vi "Matrix_Diag.vi"(11 "input matrix":T1) -> (3 "output matrix":T1)   [LabVIEW 2019, in "Trajectory_Library.lvlib"]
doc: "Returns the diagonal elements inside a vector or square matrix.\n \nIf \"this\" Matrix is a vector then a square matrix is returned. If a \"this\" Matrix}is a matrix then a vector of diagonal elements is returned.\n \n\nInputs:\n - input matrix -- The input matrix\n\nOutputs:\n - output matrix -- The diagonal elements inside a vector or a square matrix."
uses:
  Trajectory_Library.lvlib
  <vilib>/Analysis/Matrix/Datatypes/RealMatrix.ctl
  <vilib>/Analysis/Matrix/NI_Matrix.lvlib
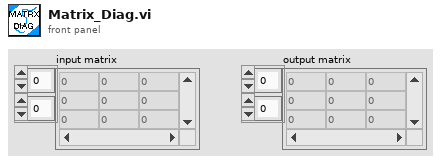
[diagram p1: front panel]
types:
  T1 = typedef "NI_Matrix.lvlib/RealMatrix.ctl" = dbl[][]
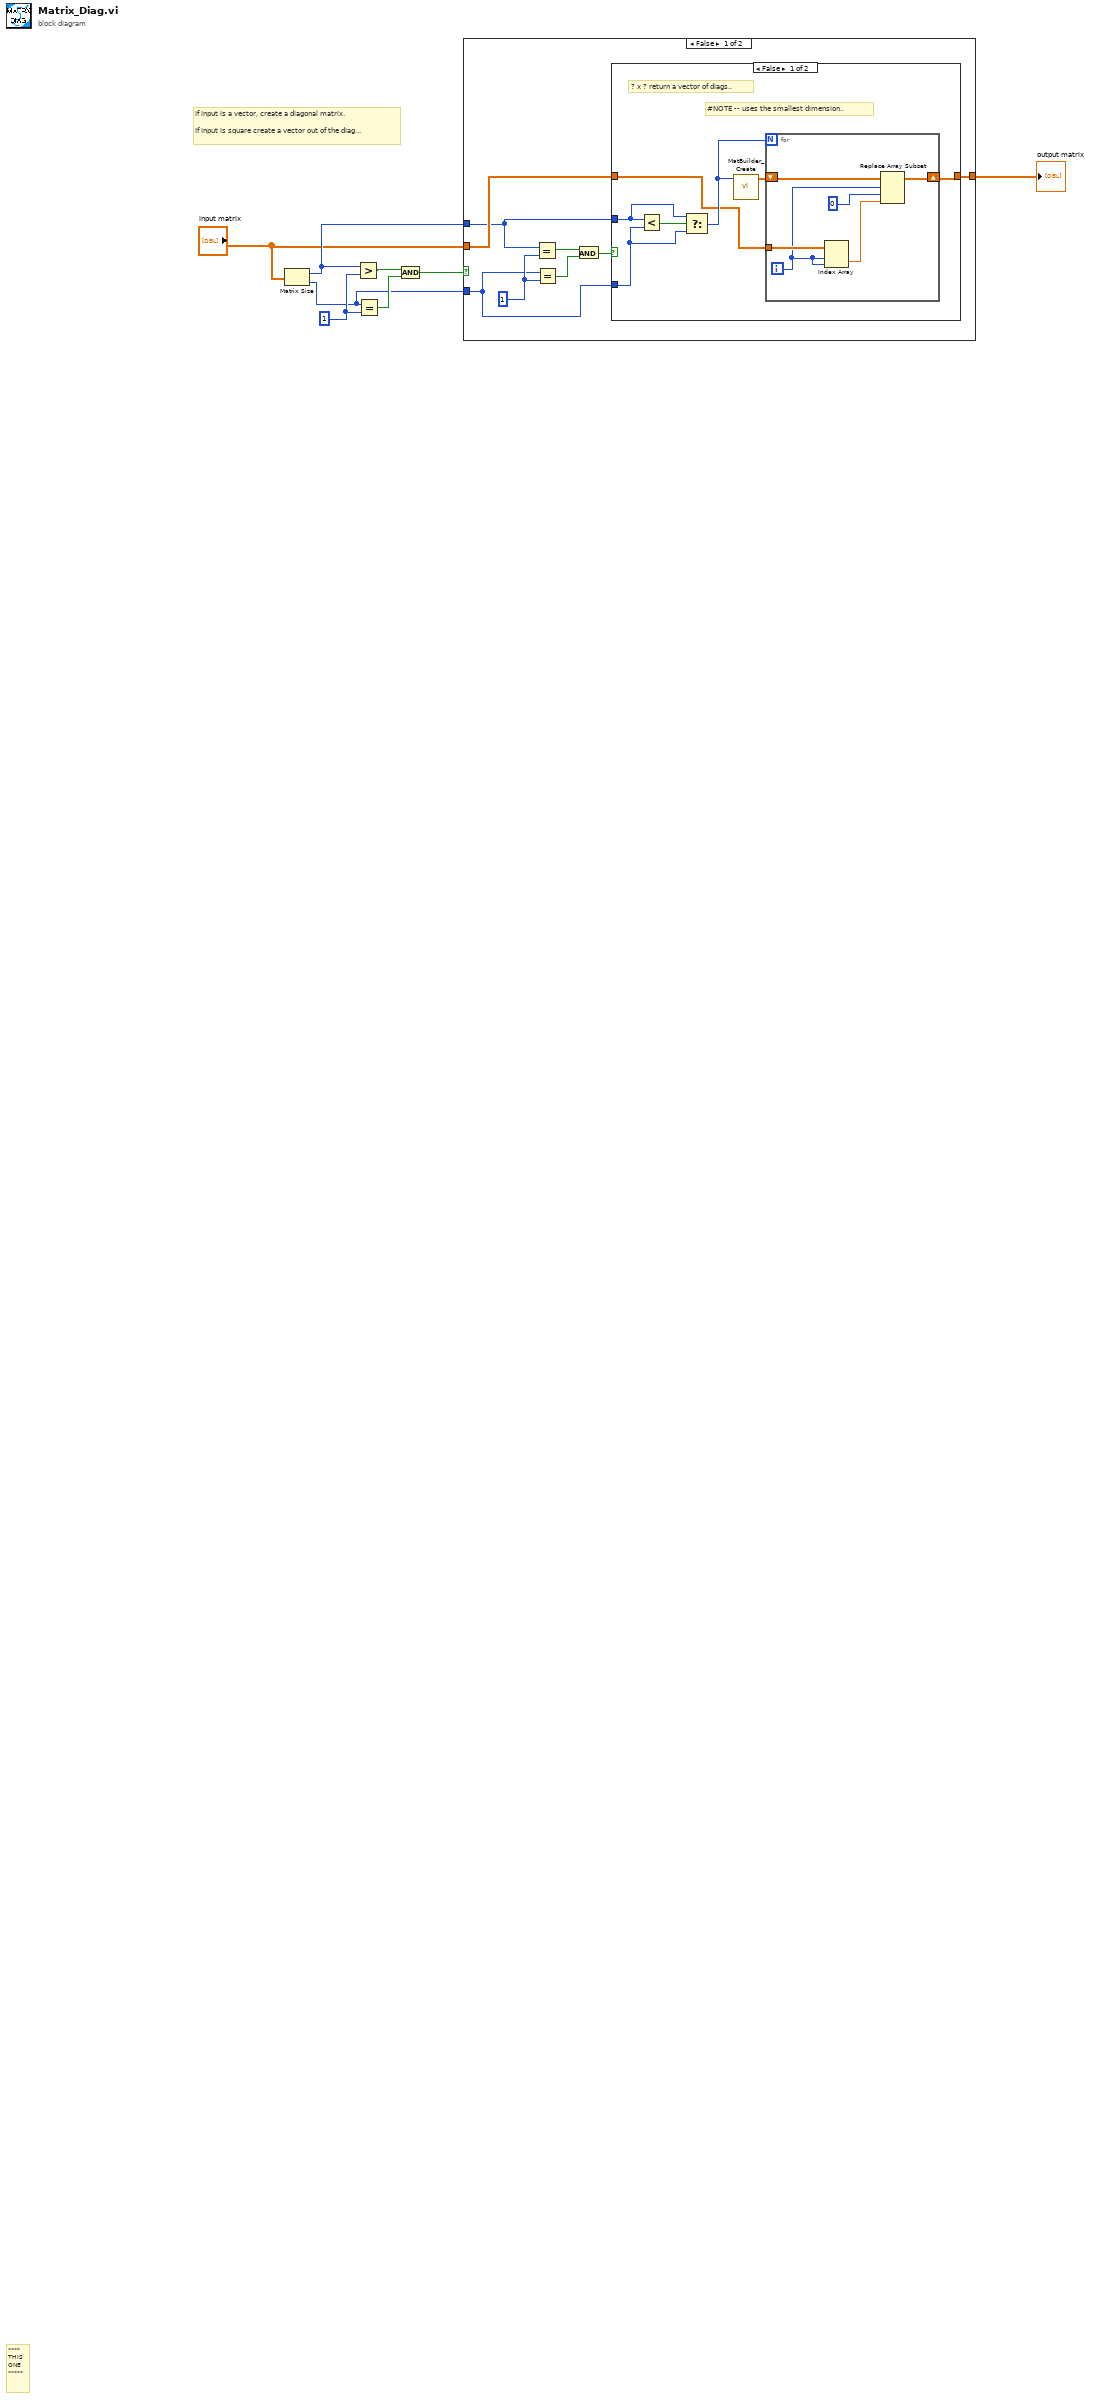
[diagram p0: block diagram]
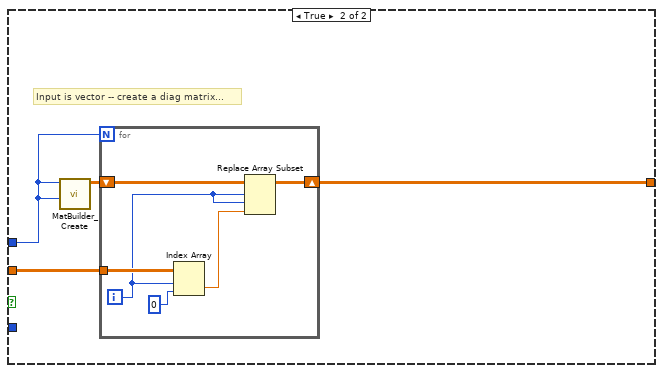
[diagram p3: hidden frame]
diagram:
  w8 = 1 ("y")
  # "If input is a vector, create a diagonal matrix.  \n\nIf input is square create a vector out of the diag..."
  # "****\nTHIS\nONE\n*****"
  n1 = Matrix Size(0:"input matrix") -> (1:w4:i32, 2:w1:i32)
  n2 = Greater?(x=w4, y=w8) -> (0:w7:bool)
  n3 = Equal?(x=w1, y=w8) -> (x = y?=w6:bool)
  n4 = And(x=w7, y=w6) -> (x .and. y?=w5:bool)
  n5 = case shown="False" w5 {
    tunnel: w4 -> [w10 w33]
    tunnel: "input matrix" -> [w12 w34]
    tunnel: [w11 w31] -> w2
    tunnel: w1 -> [w9 _]
    frame False {
      w16 = 1 ("y")
      n6 = Equal?(x=w10, y=w16) -> (x = y?=w15:bool)
      n7 = Equal?(x=w9, y=w16) -> (x = y?=w14:bool)
      n8 = And(x=w15, y=w14) -> (x .and. y?=w13:bool)
      n9 = case shown="False" w13 {
        tunnel: w12 -> [w18 w30]
        tunnel: [w17 w30] -> w11
        tunnel: w10 -> [w22 _]
        tunnel: w9 -> [w21 _]
        frame False {
          # "#NOTE -- uses the smallest dimension.."
          # "? x ? return a vector of diags.."
          n10 = Less?(x=w22, y=w21) -> (x < y?=w23:bool)
          n11 = Select(t=w22, s=w23, f=w21) -> (s? t:f=w19:i32)
          n12 = call "MatBuilder_Create.vi"("Rows"=w19) -> ("output matrix"=w20:T1)  [unwired: 10 in]
          n13 = for {
            N: w19 -> [_]
            tunnel: w18 -> [w29]
            shift-right: [w26] -> w17
            shift-left: w20 -> [w27]
            i -> [w25]
            n14 = Index Array(array=w29, index (row)=w25, index (col)=w25) -> (element=w28:dbl)
            n15 = Replace Array Subset(array=w27, new element=w28, index (row)=w25, index (col)=0) -> (w26:T1)
          }
        }
        frame True {
          # "1 x 1 - return itself."
        }
      }
    }
    frame True {
      # "Input is vector -- create a diag matrix..."
      n16 = call "MatBuilder_Create.vi"("Columns"=w33, "Rows"=w33) -> ("output matrix"=w32:T1)  [unwired: 9 in]
      n17 = for {
        N: w33 -> [_]
        tunnel: w34 -> [w40]
        shift-right: [w35] -> w31
        shift-left: w32 -> [w36]
        i -> [w38]
        n18 = Index Array(array=w40, index (row)=w38, index (col)=0) -> (element=w37:dbl)
        n19 = Replace Array Subset(array=w36, new element=w37, index (row)=w38, index (col)=w38) -> (w35:T1)
      }
    }
  }
  "output matrix" <- w2
